vi "New Write When Visible Subscription.vi"(9 "Ctl Refnum":refnum<vi>, 10 "Ignore Past Updates? (F)":bool, 11 "WriteWhenVisibleSubscription In":refnum<class "WriteWhenVisibleSubscription.lvclass">) -> (3 "WriteWhenVisibleSubscription Out":refnum<class "WriteWhenVisibleSubscription.lvclass">)   [LabVIEW 2018, in "MVA Framework.lvlib" / "SubscriptionPolicy.lvlib" / "WriteWhenVisibleSubscription.lvclass"]
doc: "新建可见时写入订阅"
uses:
  WriteWhenVisibleSubscription.lvclass
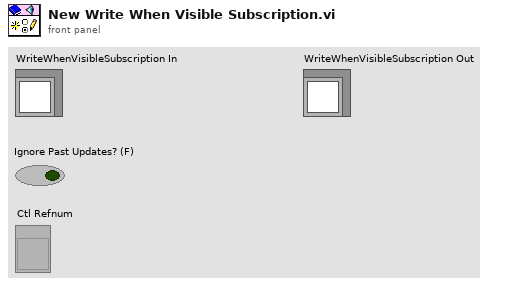
[diagram p1: front panel]
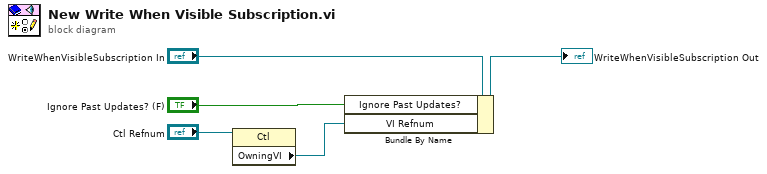
[diagram p0: block diagram]
diagram:
  n1 = property class="Ctl"(reference="Ctl Refnum") -> ("OwningVI"=w1:refnum<vi>)  [unwired: 1 in, 2 out]
  n2 = Bundle By Name(cluster="WriteWhenVisibleSubscription In", "Ignore Past Updates?"="Ignore Past Updates? (F)", "VI Refnum"=w1) -> (→"WriteWhenVisibleSubscription Out":refnum<class "WriteWhenVisibleSubscription.lvclass">)
